vi "KH monitor.vi"() -> ()   [LabVIEW 2013]
uses:
  Lock-in Globals Multiple Inputs and Outputs.vi
panel:
  out "CH8":dbl(graph)
  in  "path":path=path "C:/"
  in  "filename":string="filename"
  out "CH7":dbl(graph)
  out "CH5":dbl(graph)
  out "CH4":dbl(graph)
  out "CH3":dbl(graph)
  out "CH2":dbl(graph)
  out "CH1":dbl(graph)
  in  "Stop Button":bool
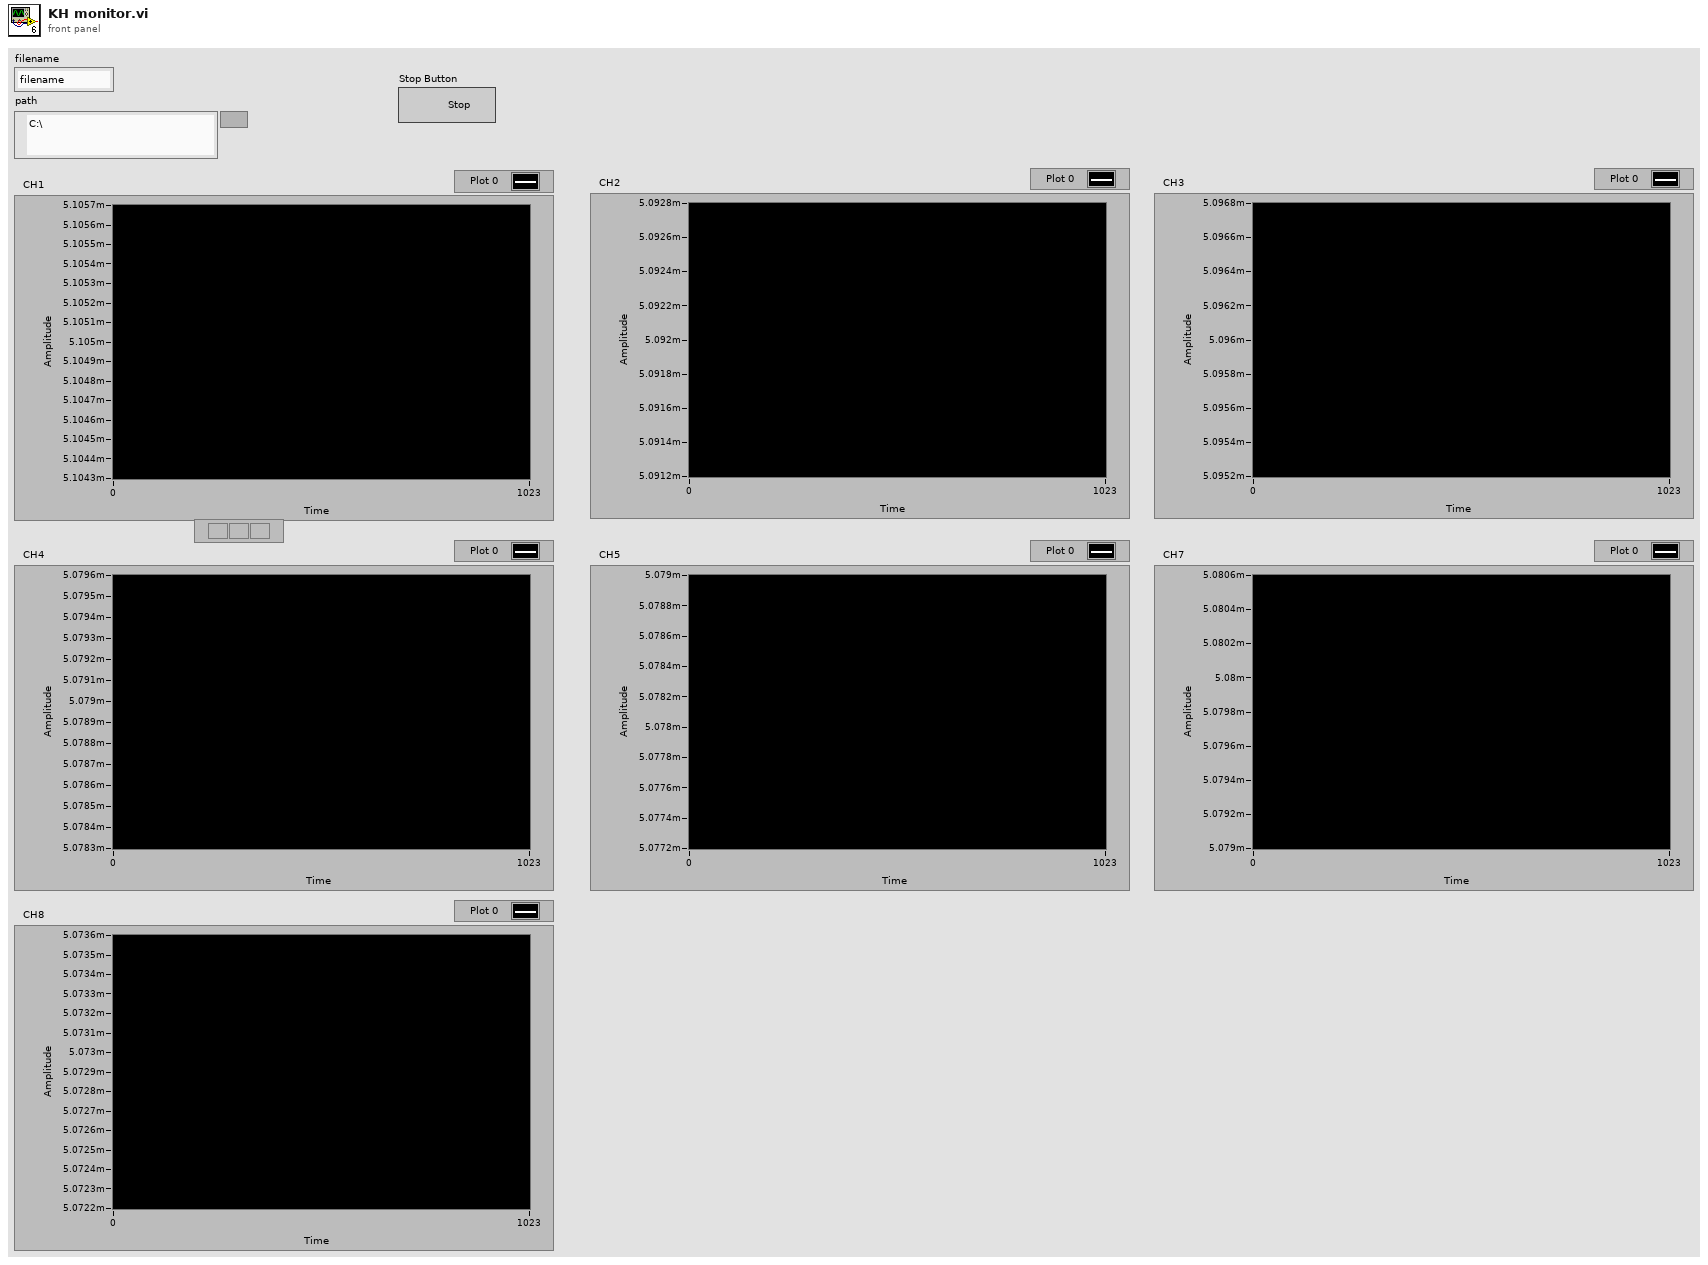
[diagram p1: front panel]
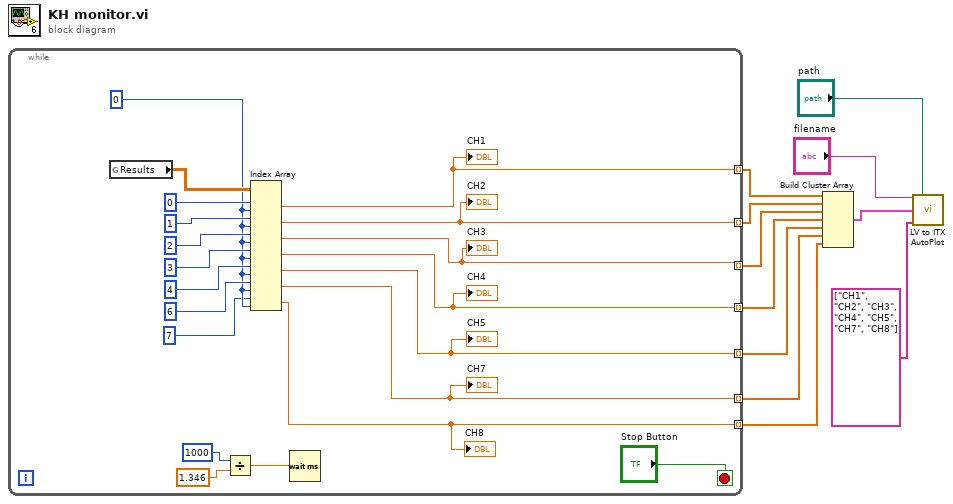
[diagram p0: block diagram]
diagram:
  n1 = while {
    tunnel: [w17] -> w11 mode=indexing
    tunnel: [w16] -> w10 mode=indexing
    tunnel: [w18] -> w9 mode=indexing
    tunnel: [w19] -> w8 mode=indexing
    tunnel: [w20] -> w7 mode=indexing
    tunnel: [w21] -> w6 mode=indexing
    tunnel: [w12] -> w1 mode=indexing
    stop <- "Stop Button" stop-if-true
    w14 = 0 ("disabled index (col)")
    n2 = global read "Lock-in Globals Multiple Inputs and Outputs.vi" "Results"() -> (w31:dbl[][])
    n3 = Divide(x=1000, y=1.346) -> (x/y=w27:dbl)
    n4 = Index Array(array=w31, index (row) #1=0 ("disabled index (col)"), index (col) #1=w14, index (row) #2=1 ("disabled index (col)"), index (col) #2=w14, index (row) #3=2 ("disabled index (col)"), index (col) #3=w14, index (row) #4=3 ("disabled index (col)"), index (col) #4=w14, index (row) #5=4 ("disabled index (col)"), index (col) #5=w14, index (row) #6=6 ("disabled index (col)"), index (col) #6=w14, index (row) #7=7 ("disabled index (col)"), index (col) #7=w14) -> (element #1=w17:dbl, element #2=w16:dbl, element #3=w18:dbl, element #4=w19:dbl, element #5=w20:dbl, element #6=w21:dbl, element #7=w12:dbl)
    "CH1" <- w17
    "CH2" <- w16
    "CH3" <- w18
    "CH4" <- w19
    "CH5" <- w20
    "CH7" <- w21
    "CH8" <- w12
    n5 = Wait (ms)(milliseconds to wait=w27) -> ()  [unwired: 1 out]
  }
  n6 = Build Cluster Array(w11, w10, w9, w8, w7, w6, w1) -> (w5:cluster{dbl[]}[])
  n7 = call <userlib>:"LV to ITX AutoPlot.vi"("filename"="filename", "path"="path", "Data"=w5, "wavenames (.Vx, etc)"=string[] ["CH1", "CH2", "CH3", "CH4", "CH5", "CH7", "CH8"]) -> ()  [unwired: 11 in, 1 out]
